vi "Labview_forward_pass.vi"() -> ()   [LabVIEW 2020]
uses:
  <vilib>/Analysis/baseanly.llb/Vector x A.vi
  <vilib>/Analysis/baseanly.llb/Real Dot Product.vi
  <vilib>/Analysis/Matrix/Numeric/Conversions/Array To Matrix - RA2.vi
  <vilib>/Analysis/NI_AALBase.lvlib
  <vilib>/Analysis/Matrix/NI_Matrix.lvlib
panel:
  out "i":i32
  out "xx size":i32
  out "xx":dbl[](array[numeric])
  out "element out":dbl
  out "XY Graph 2":cluster{i32[], dbl[]}(graph)
  out "y":dbl
  out "Array":i32[](array[numeric])
  out "XY Graph":T1(graph)
  out "X":dbl[](graph)
  out "Waveform Graph":waveform(dbl)(graph)
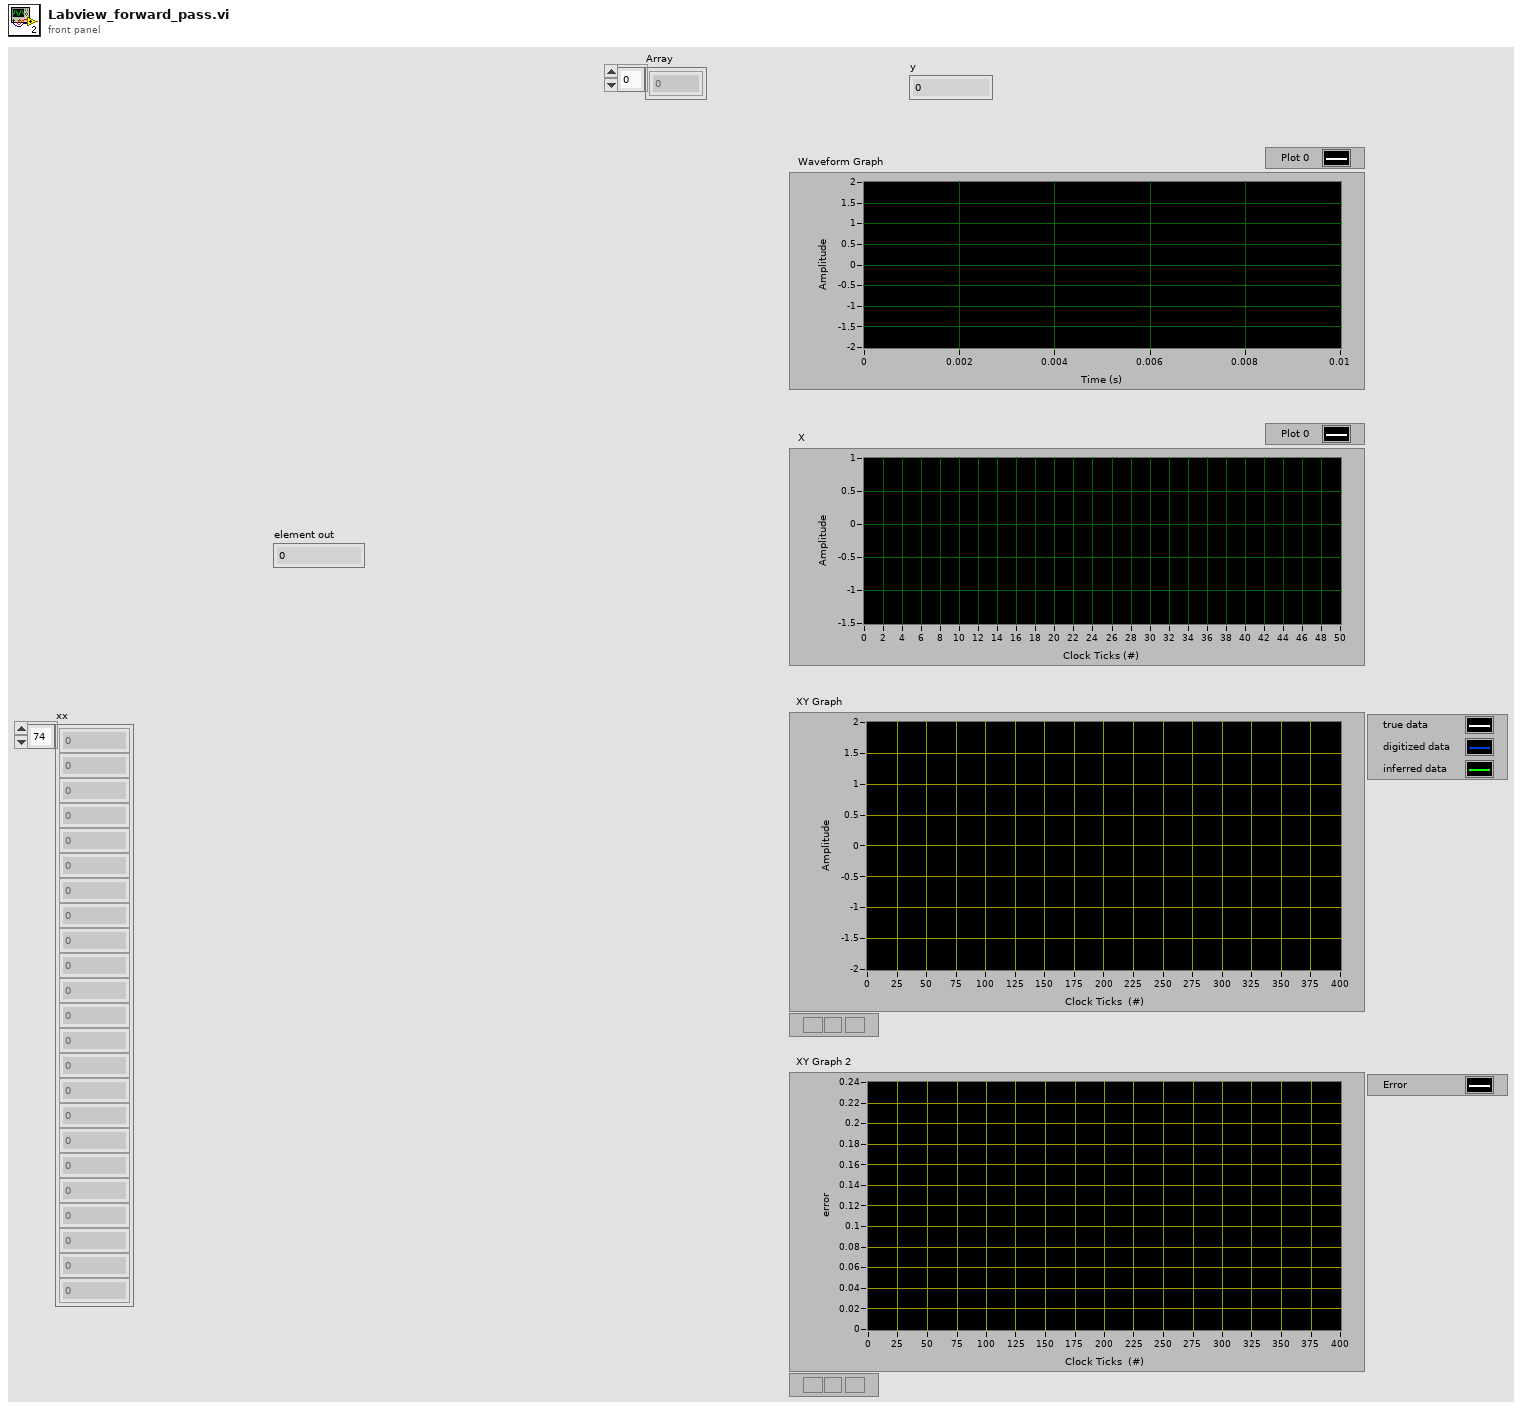
[diagram p1: front panel]
types:
  T1 = cluster{i32[], "array type (2D Dbl) out":dbl[]}[]
  T2 = typedef "NI_Matrix.lvlib/RealMatrix.ctl" = dbl[][]
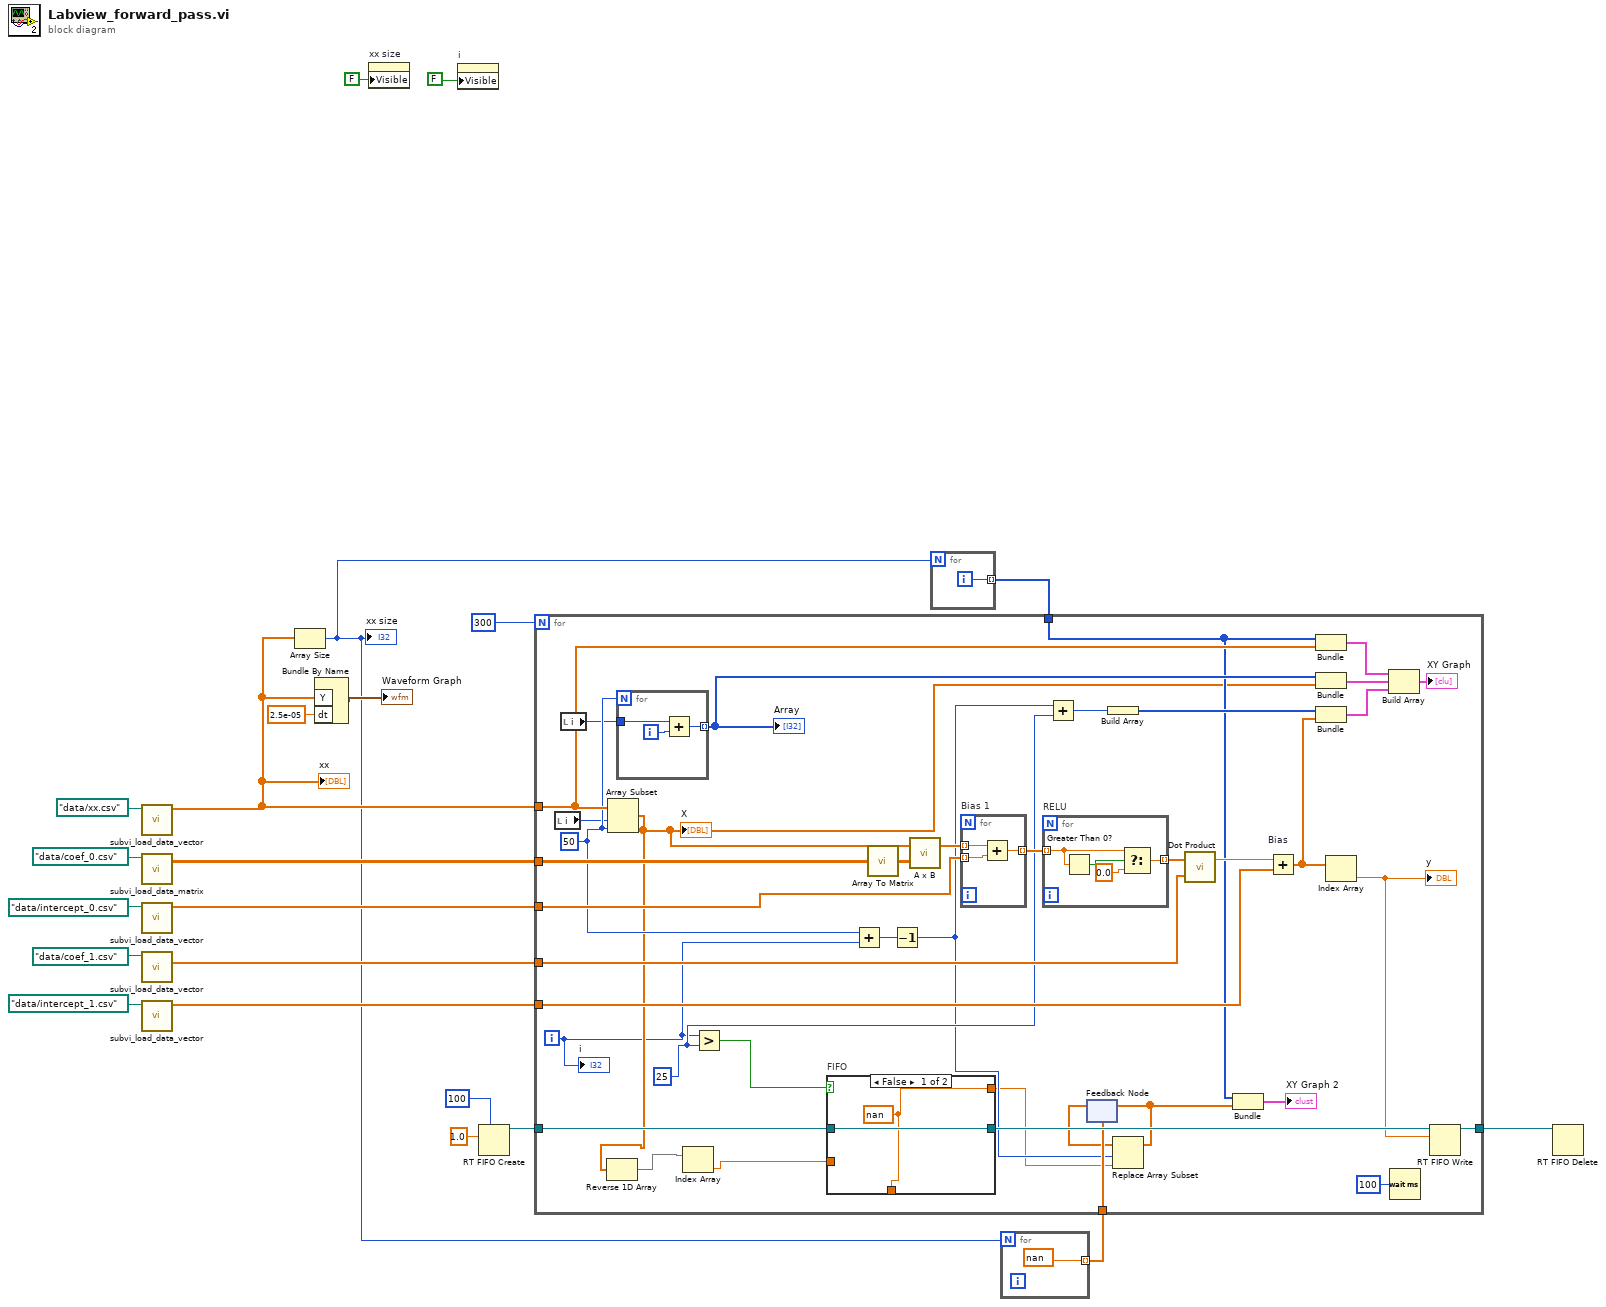
[diagram p0: block diagram]
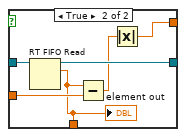
[diagram p2: hidden frame]
diagram:
  n1 = call "subvi_load_data_vector.vi"("default name"=path "data/xx.csv") -> ("array type (2D Dbl) out"=w7:dbl[])  [unwired: 10 in]
  "xx" <- w7
  n2 = call "subvi_load_data_matrix.vi"("default name"=path "data/coef_0.csv") -> ("array"=w12:dbl[][])  [unwired: 10 in]
  n3 = call "subvi_load_data_vector.vi"("default name"=path "data/intercept_0.csv") -> ("array type (2D Dbl) out"=w15:dbl[])  [unwired: 10 in]
  n4 = call "subvi_load_data_vector.vi"("default name"=path "data/coef_1.csv") -> ("array type (2D Dbl) out"=w16:dbl[])  [unwired: 10 in]
  n5 = call "subvi_load_data_vector.vi"("default name"=path "data/intercept_1.csv") -> ("array type (2D Dbl) out"=w14:dbl[])  [unwired: 10 in]
  n6 = Array Size(array=w7) -> (size(s)=w1:i32)
  "xx size" <- w1
  n7 = Bundle By Name("Y"=w7, "dt"=2.5e-05) -> (→"Waveform Graph":waveform(dbl))  [unwired: 1 in]
  n8 = property on="xx size" class="DigNum (strict)"("Visible"=FALSE) -> ()  [unwired: 2 in, 2 out]
  n9 = property on="i" class="DigNum (strict)"("Visible"=FALSE) -> ()  [unwired: 2 in, 2 out]
  n10 = RT FIFO Create(1:1.0 ("dt"), 4:u32 100 ("size (10)")) -> (8:w3:refnum<k33>)  [unwired: 6 in, 2 out]
  n11 = for {
    N: w1 -> [_]
    tunnel: [w23] -> w10 mode=indexing
    i -> [w23]
  }
  n12 = for {
    N: w1 -> [_]
    tunnel: [nan] -> w8 mode=indexing
  }
  n13 = for {
    N: 300 -> [_]
    tunnel: w16 -> [w59]
    tunnel: w15 -> [w58]
    tunnel: w14 -> [w57]
    tunnel: w12 -> [w56]
    tunnel: w7 -> [w52]
    tunnel: w10 -> [w41]
    tunnel: w3 -> [w45]
    tunnel: [w43] -> w4
    tunnel: w8 -> [w39]
    i -> [w26]
    w35 = 25 ("y")
    w36 = 50 ("length")
    n14 = local read "i"() -> (w25:i32)
    n15 = local read "i"() -> (w27:i32)
    n16 = Array Subset(array=w52, index=w25, length=w36) -> (w32:dbl[])
    "X" <- w32
    n17 = Reverse 1D Array(array=w32) -> (reversed array=w31:dbl[])
    n18 = for {
      N: w36 -> [_]
      tunnel: w27 -> [w74]
      tunnel: [w73] -> w55 mode=indexing
      i -> [w75]
      n19 = Add(x=w74, y=w75) -> (x+y=w73:i32)
    }
    "Array" <- w55
    n20 = Index Array(array=w31) -> (element=w30:dbl)  [unwired: 1 in]
    n21 = Greater?(x=w26, y=w35) -> (0:w44:bool)
    n22 = case "FIFO" shown="False" w44 {
      tunnel: w45 -> [w66 w72]
      tunnel: [w66 w71] -> w42
      tunnel: [w65 w70] -> w28
      tunnel: w30 -> [_ w68]
      tunnel: [w65 w67] -> _
      frame False {
        w65 = nan
      }
      frame True {
        n23 = RT FIFO Read(0:w72) -> (8:w71:refnum<k33>, 9:w67:dbl)  [unwired: 3 in, 3 out]
        "element out" <- w67
        n24 = Subtract(x=w67, y=w68) -> (x-y=w69:dbl)
        n25 = Absolute Value(x=w69) -> (abs(x)=w70:dbl)
      }
    }
    n26 = Add(x=w36, y=w26) -> (x+y=w34:i32)
    n27 = call-poly <vilib>:"Array To Matrix.vi"("Real 2D Array"=w56) -> ("Real Matrix"=w62:T2)
    n28 = Decrement(x=w34) -> (x-1=w33:i32)
    n29 = call-poly <vilib>:"A x B.vi"("Matrix A"=w62, "Vector V'"=w32) -> ("V' x A"=w64:dbl[])  [unwired: 1 out]
    n30 = for "Bias 1" {
      tunnel: w64 -> [w82] mode=indexing
      tunnel: [w81] -> w63 mode=indexing
      tunnel: w58 -> [w80] mode=indexing
      n31 = Add(x=w82, y=w80) -> (x+y=w81:dbl)
    }
    n32 = for "RELU" {
      tunnel: w63 -> [w79] mode=indexing
      tunnel: [w78] -> w61 mode=indexing
      n33 = Greater Than 0?(x=w79) -> (x > 0?=w76:bool)
      n34 = Select(t=w79, s=w76, f=0.0) -> (s? t:f=w78:dbl)
    }
    n35 = Add(x=w33, y=w35) -> (x+y=w50:i32)
    n36 = feedback #1(w39) -> (w37:dbl[])
    n37 = Build Array(w50) -> (w49:i32[])
    n38 = Replace Array Subset(array=w37, new element=w28, index=w33) -> (w38:dbl[])
    n39 = feedback-in #1(w38) -> ()
    n40 = call-poly <vilib>:"Dot Product.vi"("Y Vector"=w59, "X Vector"=w61) -> ("X * Y"=w60:dbl)  [unwired: 1 out]
    n41 = Bundle(w41, w38) -> (→"XY Graph 2":cluster{i32[], dbl[]})  [unwired: 1 in]
    n42 = Add "Bias"(x=w60, y=w57) -> (x+y=w51:dbl[])
    n43 = Bundle(w41, "array type (2D Dbl) out"=w52) -> (w46:cluster{i32[], "array type (2D Dbl) out":dbl[]})  [unwired: 1 in]
    n44 = Bundle(w55, w32) -> (w54:cluster{i32[], dbl[]})  [unwired: 1 in]
    n45 = Bundle(w49, w51) -> (w47:cluster{i32[], dbl[]})  [unwired: 1 in]
    n46 = Index Array(array=w51) -> (element=w29:dbl)  [unwired: 1 in]
    "y" <- w29
    n47 = Build Array(w46, w54, w47) -> (→"XY Graph":T1)
    n48 = Wait (ms)(milliseconds to wait=u32 100) -> ()  [unwired: 1 out]
    n49 = RT FIFO Write(0:w42, 1:w29) -> (8:w43:refnum<k33>)  [unwired: 3 in, 3 out]
    "i" <- w26
  }
  n50 = RT FIFO Delete(0:w4) -> ()  [unwired: 2 in, 1 out]
